vi "Create Result Row.vi"(10 "Values":refnum<class "Type.lvclass">[](array[class]), 11 "Database in":refnum<class "Database Platform.lvclass">) -> (1 "Result":refnum<class "Result Row.lvclass">, 3 "Database out":refnum<class "Database Platform.lvclass">)   [LabVIEW 2020, in "Conditu2.lvlib" / "Database Platform.lvclass"]
uses:
  Database Platform.lvclass
  Columns/Type/Type.lvclass
  Result Row/Result Row.lvclass
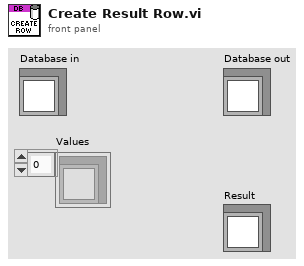
[diagram p1: front panel]
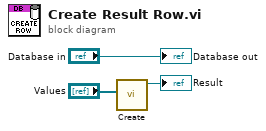
[diagram p0: block diagram]
diagram:
  n1 = call "Create.vi"("Values"="Values") -> ("Result Row out"=→"Result":refnum<class "Result Row.lvclass">)  [unwired: 8 in, 2 out]
  "Database out" <- "Database in"
